vi "Read Actor DVR.vi"(11 "TEMPLATE Actor in":refnum<class "TEMPLATE Actor.lvclass">) -> (2 "Actor DVR":refnum<data-value>)   [LabVIEW 2020, in "_Template.lvlib" / "Templates.lvlib" / "TEMPLATE jettl Actor.lvlib" / "TEMPLATE Actor.lvlib" / "TEMPLATE Actor.lvclass"]
uses:
  jettl/jettl/Msg/Msg.lvclass
  jettl/jettl/Refs/Refs.lvclass
  TEMPLATE Actor.lvclass
  TEMPLATE Actor.lvclass/TEMPLATE Actor.ctl
  jettl/jettl/Actor/Actor.lvclass
  jettl/jettl/Msg Set.ctl
  jettl/jettl/jettl.lvlib
  jettl/jettl/Actor.ctl
  jettl/jettl/Msgs.ctl
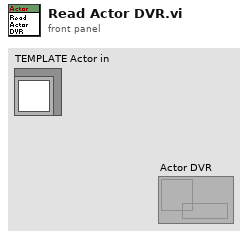
[diagram p1: front panel]
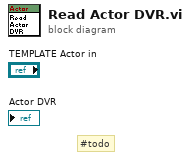
[diagram p0: block diagram]
diagram:
  # "#todo"
